vi "Remove Sink.vi"(6 "Sink Name":string, 8 "error in (no error)":errorcluster, 11 "Application Log in":refnum<class "Application Log.lvclass">) -> (0 "error out":errorcluster, 2 "Found?":bool, 3 "Application Log out":refnum<class "Application Log.lvclass">, 4 "Log Sink":refnum<data-value>)   [LabVIEW 2016, in "Stream Log.lvlib" / "Application Log.lvclass"]
doc: "--\nCopyright © 2017 Composed SystemsI All rights reserved.\n\nAuthor: Jon McBee <jon.mcbee@composed.io>\n\nThis library is provided \"AS IS\" ,WITHOUT WARRANTIES OR\nCONDITIONS OF ANY KIND, either express or implied.\n\nComposed Systems -- composed.io\n\nStream 0.0.1.1\nJon McBee - Composed Systems\nCopyright (c) 2017, Composed Systems"
uses:
  <userlib>/Composed Systems/Stream/Log/Application Log/Application Log.lvclass
  <userlib>/Composed Systems/Stream/Log/Log Sink/Log Sink.lvclass
  <userlib>/Composed Systems/Stream/Log/Application Log/Application Log.lvclass/Application Log.ctl
  <userlib>/Composed Systems/Stream/Log/Sink Look Up Table/Sink Look Up Table.lvclass
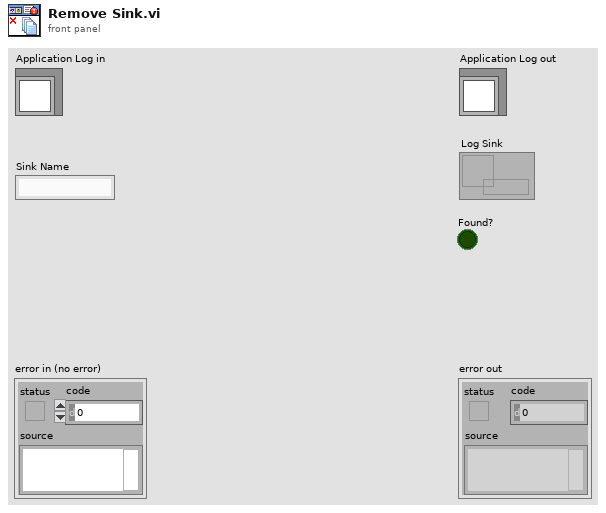
[diagram p1: front panel]
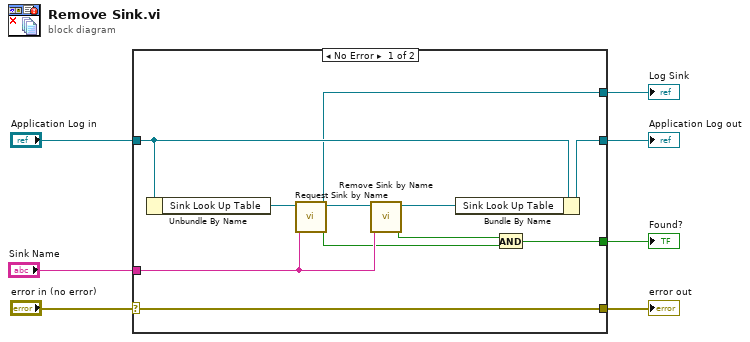
[diagram p0: block diagram]
diagram:
  n1 = case shown="No Error" "error in (no error)" {
    selector: "error in (no error)" -> [w18 w20]
    tunnel: [w18 w20] -> w6
    tunnel: [w15 w19] -> w4
    tunnel: "Application Log in" -> [w16 w19]
    tunnel: "Sink Name" -> [w12 _]
    tunnel: [w9 _] -> w2
    tunnel: [w8 _] -> w1
    frame No Error {
      n2 = Unbundle By Name(w16) -> ("Sink Look Up Table"=w14:refnum<class "Sink Look Up Table.lvclass">)
      n3 = call <userlib>:"Request Sink by Name.vi"("Sink Name"=w12, "Sink Look Up Table in"=w14) -> ("Found?"=w10:bool, "Log Sink"=w8:refnum<data-value>, "Sink Look Up Table out"=w13:refnum<class "Sink Look Up Table.lvclass">)  [unwired: 6 in, 1 out]
      n4 = call <userlib>:"Remove Sink by Name.vi"("Sink Name"=w12, "Sink Look Up Table in"=w13) -> ("Found?"=w11:bool, "Sink Look Up Table out"=w17:refnum<class "Sink Look Up Table.lvclass">)  [unwired: 7 in, 1 out]
      n5 = Bundle By Name(cluster=w16, "Sink Look Up Table"=w17) -> (w15:refnum<class "Application Log.lvclass">)
      n6 = And(x=w11, y=w10) -> (x .and. y?=w9:bool)
    }
    frame Error {
    }
  }
  "error out" <- w6
  "Application Log out" <- w4
  "Found?" <- w2
  "Log Sink" <- w1
